vi "DestroyWindowSurface.vi"(8 "No Error":errorcluster, 11 "Window [SDL_Window *]":i64 format="%.0x") -> (0 "Error Out":errorcluster)   [LabVIEW 2024, in "SDL3.lvlib" / "Video.lvlib"]
doc: "<B>Summary</B>\nDestroy the surface associated with the window."
uses:
  Video.lvlib
  Lib/SDL3.dll
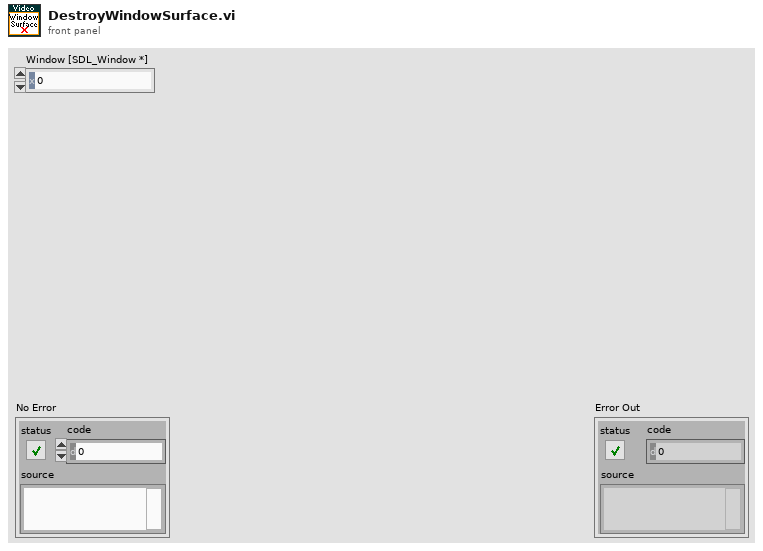
[diagram p1: front panel]
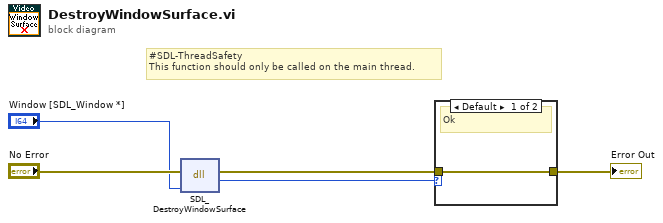
[diagram p0: block diagram]
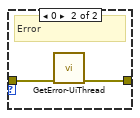
[diagram p2: hidden frame]
diagram:
  # "#SDL-ThreadSafety\nThis function should only be called on the main thread."
  n1 = dll-call lib="C:/Users/Thomas/Documents/Projects/LV-SDL3/Sources/SDL3/Lib/SDL3.*" fn="SDL_DestroyWindowSurface"(error in="No Error", "window"="Window [SDL_Window *]") -> (error out=w2:errorcluster, "return type"=w1:i32)  [unwired: 3 in, 1 out]
  n2 = case shown="Default" w1 {
    tunnel: w2 -> [w6 w8]
    tunnel: [w6 w7] -> w4
    frame Default {
      # "Ok"
    }
    frame 0 {
      # "Error"
      n3 = call "GetError-UiThread.vi"("No Error"=w8) -> ("error out"=w7:errorcluster)  [unwired: 10 in]
    }
  }
  "Error Out" <- w4
